vi "subAxisParamEx.vi"(1 "AxisId":i32=1, 2 "Index":i32=1) -> ()   [LabVIEW 2020]
panel:
  in  "SetOne":bool
  in  "PwmFreq":u16(ring) caption="Pwm frequency [Hz]" items=["20000", "80000"]
  in  "EncLines":i32=500 caption="Encoder lines" min=1 max=65535
  in  "MotorCommCounts":i32=1 caption="Encoder counts per commutating cycle" min=1 max=65535
  in  "PhaseInitAmp":i32 caption="Phase init. amplitude" min=0 max=100
  in  "MotorPoles":i32=1 caption="Motor poles" min=1 max=65535
  in  "MicrostepMode":i32=1 caption="Microstep mode" min=1 max=256
  in  "HoldCur":i32 caption="Hold current [%]" min=0 max=100
  in  "BrakeDecel":dbl caption="Brake deceleration" min=0.0 format="%.3f"
  in  "Vel":dbl format="%.3f"
  in  "RefDecel":dbl caption="Deceleration" min=0.0 format="%.3f"
  in  "SlowRefVel":dbl caption="Slow velocity [mm/s]" max=16777215.0 format="%.3f"
  in  "Jerk":i32 min=0
  in  "Decel":dbl caption="Deceleration" min=0.0 format="%.3f"
  in  "PhaseInitTime":i32=1 caption="Phase init. time" min=0
  in  "DriveCur":i32 caption="Drive current [%]" min=0 max=100
  in  "MaxPosErr":i32=10000 caption="Max. pos. error [Inc]" min=0
  in  "SampleTime":i32=256 caption="Sample time [µs]" min=204 max=19968
  in  "MaxOut":i32=99 caption="Maximum output [%]" min=0 max=99
  out "SetNr":u8
  in  "KD":i32=150
  in  "I-Limit":i32=100000
  in  "KI":i32=20
  in  "D-Time":i32 caption="Time"
  in  "KP":i32=30
  in  "Accel":dbl caption="Acceleration" format="%.3f"
  in  "FastRefVel":dbl caption="Fast velocity [mm/s]" max=16777215.0 format="%.3f"
  in  "FreeVel":dbl caption="Free velocity [mm/s]" min=0.0 max=16777215.0 format="%.3f"
  in  "PosVel":dbl caption="Velocity [mm/s]" max=16777215.0 format="%.3f"
  in  "SetAll":bool
  in  "End":bool
  # "Axis"
  # "Positioning"
  # "Reference run"
  # "Limit switches"
  # "Power amplifier"
  # "Velocity mode"
  # "[mm/s]"
  # "PID regulator"
  # "Step motor data"
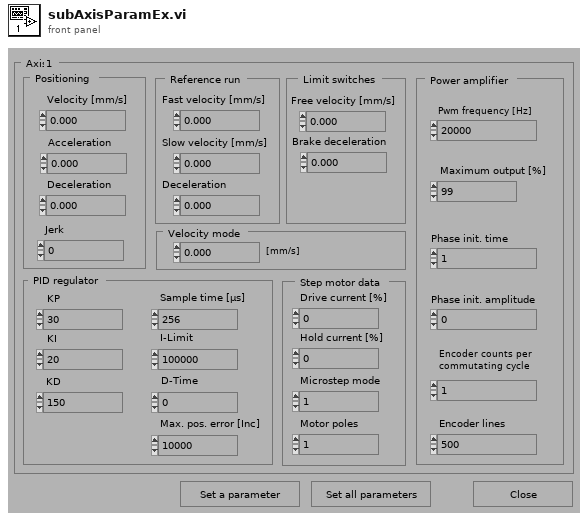
[diagram p1: front panel]
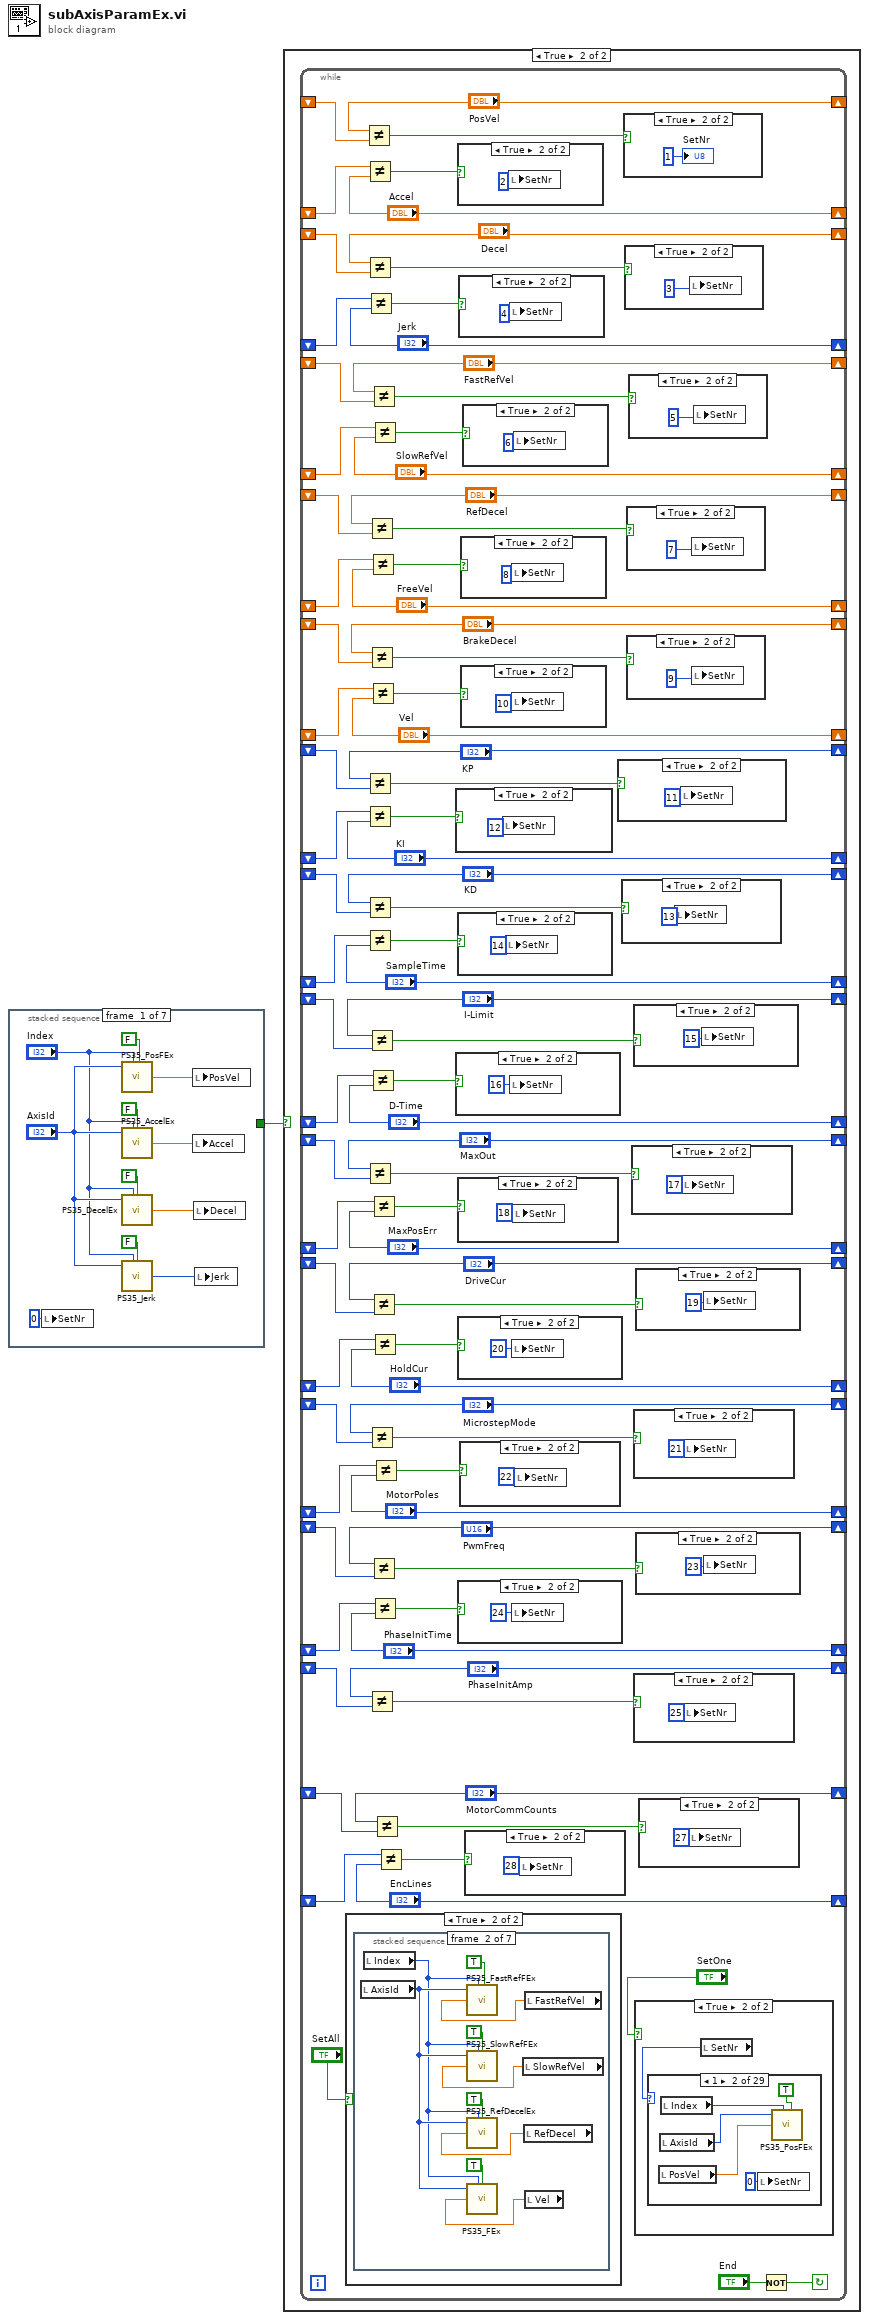
[diagram p0: block diagram]
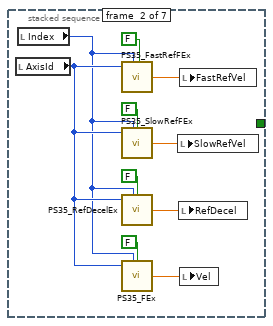
[diagram p2: hidden frame]
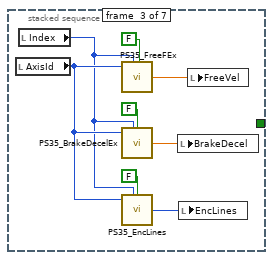
[diagram p3: hidden frame]
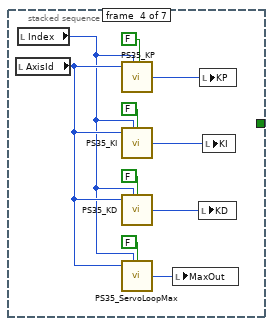
[diagram p4: hidden frame]
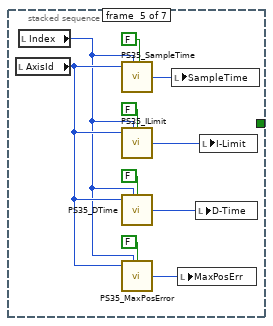
[diagram p5: hidden frame]
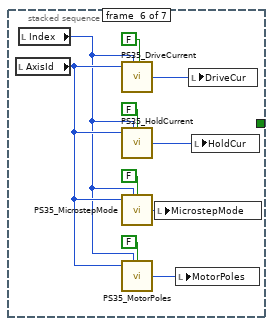
[diagram p6: hidden frame]
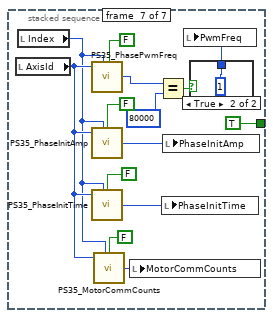
[diagram p7: hidden frame]
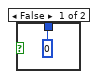
[diagram p8: hidden frame]
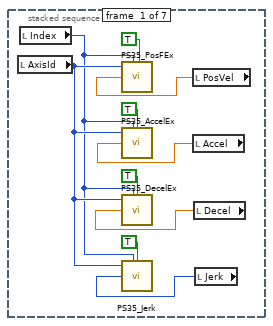
[diagram p11: hidden frame]
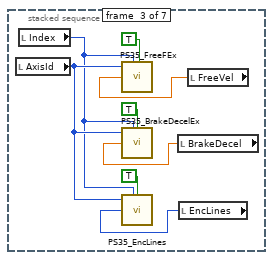
[diagram p12: hidden frame]
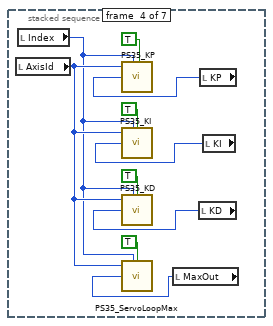
[diagram p13: hidden frame]
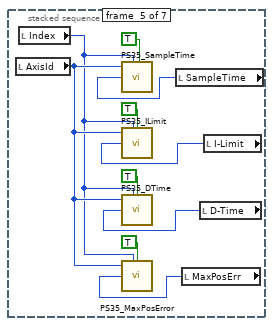
[diagram p14: hidden frame]
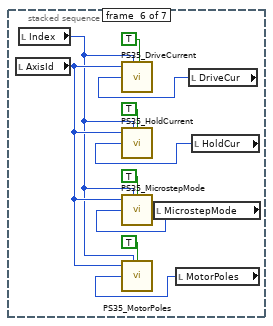
[diagram p15: hidden frame]
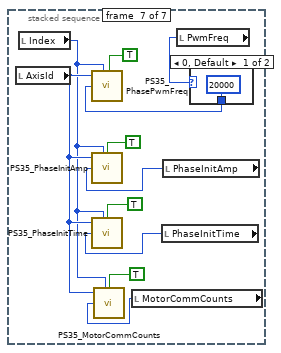
[diagram p16: hidden frame]
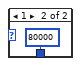
[diagram p17: hidden frame]
diagram:
  n1 = stacked-sequence {
    tunnel: [_ _ _ _ _ _ TRUE] -> w1
    frame #0 {
      n2 = local write "SetNr"(u8 0 ("SetNr")) -> ()
      n3 = call "PS35_PosFEx.vi"("Axis number"="AxisId", "Control unit ID"="Index", "function"=FALSE ("WriteRead")) -> ("dValue-Out"=w10:dbl)  [unwired: 5 in, 1 out]
      n4 = call "PS35_AccelEx.vi"("Axis number"="AxisId", "Control unit ID"="Index", "function"=FALSE ("WriteRead")) -> ("dValue-Out"=w9:dbl)  [unwired: 5 in, 1 out]
      n5 = call "PS35_DecelEx.vi"("Axis number"="AxisId", "Control unit ID"="Index", "function"=FALSE ("WriteRead")) -> ("dValue-Out"=w6:dbl)  [unwired: 5 in, 1 out]
      n6 = call "PS35_Jerk.vi"("Axis number"="AxisId", "Control unit ID"="Index", "function"=FALSE ("WriteRead")) -> ("Value-Out"=w5:i32)  [unwired: 5 in, 1 out]
      n7 = local write "PosVel"(w10) -> ()
      n8 = local write "Accel"(w9) -> ()
      n9 = local write "Decel"(w6) -> ()
      n10 = local write "Jerk"(w5) -> ()
    }
    frame #1 {
      n11 = local read "AxisId"() -> (w14:i32)
      n12 = local read "Index"() -> (w13:i32)
      n13 = call "PS35_FastRefFEx.vi"("Axis number"=w14, "Control unit ID"=w13, "function"=FALSE ("WriteRead")) -> ("dValue-Out"=w21:dbl)  [unwired: 5 in, 1 out]
      n14 = call "PS35_SlowRefFEx.vi"("Axis number"=w14, "Control unit ID"=w13, "function"=FALSE ("WriteRead")) -> ("dValue-Out"=w20:dbl)  [unwired: 5 in, 1 out]
      n15 = call "PS35_RefDecelEx.vi"("Axis number"=w14, "Control unit ID"=w13, "function"=FALSE ("WriteRead")) -> ("dValue-Out"=w17:dbl)  [unwired: 5 in, 1 out]
      n16 = call "PS35_FEx.vi"("Axis number"=w14, "Control unit ID"=w13, "function"=FALSE ("WriteRead")) -> ("dValue-Out"=w16:dbl)  [unwired: 5 in, 1 out]
      n17 = local write "SlowRefVel"(w20) -> ()
      n18 = local write "RefDecel"(w17) -> ()
      n19 = local write "FastRefVel"(w21) -> ()
      n20 = local write "Vel"(w16) -> ()
    }
    frame #2 {
      n21 = local read "AxisId"() -> (w24:i32)
      n22 = local read "Index"() -> (w23:i32)
      n23 = call "PS35_FreeFEx.vi"("Axis number"=w24, "Control unit ID"=w23, "function"=FALSE ("WriteRead")) -> ("dValue-Out"=w29:dbl)  [unwired: 5 in, 1 out]
      n24 = call "PS35_BrakeDecelEx.vi"("Axis number"=w24, "Control unit ID"=w23, "function"=FALSE ("WriteRead")) -> ("dValue-Out"=w28:dbl)  [unwired: 5 in, 1 out]
      n25 = call "PS35_EncLines.vi"("Axis number"=w24, "Control unit ID"=w23, "function"=FALSE ("WriteRead")) -> ("Value-Out"=w25:i32)  [unwired: 5 in, 1 out]
      n26 = local write "BrakeDecel"(w28) -> ()
      n27 = local write "EncLines"(w25) -> ()
      n28 = local write "FreeVel"(w29) -> ()
    }
    frame #3 {
      n29 = local read "AxisId"() -> (w32:i32)
      n30 = local read "Index"() -> (w31:i32)
      n31 = call "PS35_KP.vi"("Axis number"=w32, "Control unit ID"=w31, "function"=FALSE ("WriteRead")) -> ("Value-Out"=w39:i32)  [unwired: 5 in, 1 out]
      n32 = call "PS35_KI.vi"("Axis number"=w32, "Control unit ID"=w31, "function"=FALSE ("WriteRead")) -> ("Value-Out"=w38:i32)  [unwired: 5 in, 1 out]
      n33 = call "PS35_KD.vi"("Axis number"=w32, "Control unit ID"=w31, "function"=FALSE ("WriteRead")) -> ("Value-Out"=w35:i32)  [unwired: 5 in, 1 out]
      n34 = call "PS35_ServoLoopMax.vi"("Axis number"=w32, "Control unit ID"=w31, "function"=FALSE ("WriteRead")) -> ("Value-Out"=w34:i32)  [unwired: 5 in, 1 out]
      n35 = local write "MaxOut"(w34) -> ()
      n36 = local write "KD"(w35) -> ()
      n37 = local write "KP"(w39) -> ()
      n38 = local write "KI"(w38) -> ()
    }
    frame #4 {
      n39 = local read "AxisId"() -> (w42:i32)
      n40 = local read "Index"() -> (w41:i32)
      n41 = call "PS35_SampleTime.vi"("Axis number"=w42, "Control unit ID"=w41, "function"=FALSE ("WriteRead")) -> ("Value-Out"=w49:i32)  [unwired: 5 in, 1 out]
      n42 = call "PS35_ILimit.vi"("Axis number"=w42, "Control unit ID"=w41, "function"=FALSE ("WriteRead")) -> ("Value-Out"=w48:i32)  [unwired: 5 in, 1 out]
      n43 = call "PS35_DTime.vi"("Axis number"=w42, "Control unit ID"=w41, "function"=FALSE ("WriteRead")) -> ("Value-Out"=w45:i32)  [unwired: 5 in, 1 out]
      n44 = call "PS35_MaxPosError.vi"("Axis number"=w42, "Control unit ID"=w41, "function"=FALSE ("WriteRead")) -> ("Value-Out"=w44:i32)  [unwired: 5 in, 1 out]
      n45 = local write "SampleTime"(w49) -> ()
      n46 = local write "MaxPosErr"(w44) -> ()
      n47 = local write "D-Time"(w45) -> ()
      n48 = local write "I-Limit"(w48) -> ()
    }
    frame #5 {
      n49 = local read "AxisId"() -> (w52:i32)
      n50 = local read "Index"() -> (w51:i32)
      n51 = call "PS35_DriveCurrent.vi"("Axis number"=w52, "Control unit ID"=w51, "function"=FALSE ("WriteRead")) -> ("Value-Out"=w59:i32)  [unwired: 5 in, 1 out]
      n52 = call "PS35_HoldCurrent.vi"("Axis number"=w52, "Control unit ID"=w51, "function"=FALSE ("WriteRead")) -> ("Value-Out"=w58:i32)  [unwired: 5 in, 1 out]
      n53 = call "PS35_MicrostepMode.vi"("Axis number"=w52, "Control unit ID"=w51, "function"=FALSE ("WriteRead")) -> ("Value-Out"=w55:i32)  [unwired: 5 in, 1 out]
      n54 = call "PS35_MotorPoles.vi"("Axis number"=w52, "Control unit ID"=w51, "function"=FALSE ("WriteRead")) -> ("Value-Out"=w54:i32)  [unwired: 5 in, 1 out]
      n55 = local write "MicrostepMode"(w55) -> ()
      n56 = local write "MotorPoles"(w54) -> ()
      n57 = local write "DriveCur"(w59) -> ()
      n58 = local write "HoldCur"(w58) -> ()
    }
    frame #6 {
      n59 = local read "AxisId"() -> (w62:i32)
      n60 = local read "Index"() -> (w61:i32)
      n61 = call "PS35_PhasePwmFreq.vi"("Axis number"=w62, "Control unit ID"=w61, "function"=FALSE ("WriteRead")) -> ("Value-Out"=w66:i32)  [unwired: 5 in, 1 out]
      n62 = call "PS35_PhaseInitAmp.vi"("Axis number"=w62, "Control unit ID"=w61, "function"=FALSE ("WriteRead")) -> ("Value-Out"=w73:i32)  [unwired: 5 in, 1 out]
      n63 = call "PS35_PhaseInitTime.vi"("Axis number"=w62, "Control unit ID"=w61, "function"=FALSE ("WriteRead")) -> ("Value-Out"=w70:i32)  [unwired: 5 in, 1 out]
      n64 = call "PS35_MotorCommCounts.vi"("Axis number"=w62, "Control unit ID"=w61, "function"=FALSE ("WriteRead")) -> ("Value-Out"=w67:i32)  [unwired: 5 in, 1 out]
      n65 = local write "MotorCommCounts"(w67) -> ()
      n66 = Equal?(x=w66, y=80000) -> (x = y?=w64:bool)
      n67 = local write "PhaseInitTime"(w70) -> ()
      n68 = local write "PhaseInitAmp"(w73) -> ()
      n69 = case shown="True" w64 {
        tunnel: [0 1] -> w63
        frame False {
        }
        frame True {
        }
      }
      n70 = local write "PwmFreq"(w63) -> ()
    }
  }
  n71 = case shown="True" w1 {
    frame False {
    }
    frame True {
      n72 = while {
        shift-left: _ -> [w81]
        shift-right: ["EncLines"] -> _
        shift-left: _ -> [w83]
        shift-right: ["MotorCommCounts"] -> _
        shift-left: _ -> [w88]
        shift-right: ["PhaseInitTime"] -> _
        shift-left: _ -> [w90]
        shift-right: ["PwmFreq"] -> _
        shift-left: _ -> [w91]
        shift-right: ["PhaseInitAmp"] -> _
        shift-left: _ -> [w103]
        shift-right: ["HoldCur"] -> _
        shift-left: _ -> [w101]
        shift-right: ["DriveCur"] -> _
        shift-left: _ -> [w98]
        shift-right: ["MotorPoles"] -> _
        shift-left: _ -> [w100]
        shift-right: ["MicrostepMode"] -> _
        shift-left: _ -> [w114]
        shift-right: ["BrakeDecel"] -> _
        shift-left: _ -> [w116]
        shift-right: ["Vel"] -> _
        shift-left: _ -> [w123]
        shift-right: ["RefDecel"] -> _
        shift-left: _ -> [w121]
        shift-right: ["FreeVel"] -> _
        shift-left: _ -> [w126]
        shift-right: ["FastRefVel"] -> _
        shift-left: _ -> [w128]
        shift-right: ["SlowRefVel"] -> _
        shift-left: _ -> [w133]
        shift-right: ["Decel"] -> _
        shift-left: _ -> [w131]
        shift-right: ["Jerk"] -> _
        shift-left: _ -> [w138]
        shift-right: ["PosVel"] -> _
        shift-left: _ -> [w142]
        shift-right: ["D-Time"] -> _
        shift-left: _ -> [w144]
        shift-right: ["I-Limit"] -> _
        shift-left: _ -> [w148]
        shift-right: ["MaxPosErr"] -> _
        shift-left: _ -> [w146]
        shift-right: ["MaxOut"] -> _
        shift-left: _ -> [w151]
        shift-right: ["SampleTime"] -> _
        shift-left: _ -> [w153]
        shift-right: ["KD"] -> _
        shift-left: _ -> [w156]
        shift-right: ["KI"] -> _
        shift-left: _ -> [w154]
        shift-right: ["KP"] -> _
        shift-left: _ -> [w159]
        shift-right: ["Accel"] -> _
        stop <- w161 continue-if-true
        n73 = case shown="True" "SetAll" {
          frame False {
          }
          frame True {
            n74 = stacked-sequence {
              frame #0 {
                n75 = local read "AxisId"() -> (w164:i32)
                n76 = local read "Index"() -> (w162:i32)
                n77 = local read "PosVel"() -> (w167:dbl)
                n78 = call "PS35_PosFEx.vi"("Axis number"=w164, "Control unit ID"=w162, "dValue-In"=w167, "function"=TRUE ("WriteRead")) -> ()  [unwired: 4 in, 2 out]
                n79 = local read "Accel"() -> (w166:dbl)
                n80 = call "PS35_AccelEx.vi"("Axis number"=w164, "Control unit ID"=w162, "dValue-In"=w166, "function"=TRUE ("WriteRead")) -> ()  [unwired: 4 in, 2 out]
                n81 = local read "Decel"() -> (w165:dbl)
                n82 = call "PS35_DecelEx.vi"("Axis number"=w164, "Control unit ID"=w162, "dValue-In"=w165, "function"=TRUE ("WriteRead")) -> ()  [unwired: 4 in, 2 out]
                n83 = local read "Jerk"() -> (w163:i32)
                n84 = call "PS35_Jerk.vi"("Axis number"=w164, "Control unit ID"=w162, "Value-In"=w163, "function"=TRUE ("WriteRead")) -> ()  [unwired: 4 in, 2 out]
              }
              frame #1 {
                n85 = local read "AxisId"() -> (w177:i32)
                n86 = local read "Index"() -> (w172:i32)
                n87 = local read "SlowRefVel"() -> (w175:dbl)
                n88 = call "PS35_SlowRefFEx.vi"("Axis number"=w177, "Control unit ID"=w172, "dValue-In"=w175, "function"=TRUE ("WriteRead")) -> ()  [unwired: 4 in, 2 out]
                n89 = local read "RefDecel"() -> (w174:dbl)
                n90 = call "PS35_RefDecelEx.vi"("Axis number"=w177, "Control unit ID"=w172, "dValue-In"=w174, "function"=TRUE ("WriteRead")) -> ()  [unwired: 4 in, 2 out]
                n91 = local read "FastRefVel"() -> (w176:dbl)
                n92 = call "PS35_FastRefFEx.vi"("Axis number"=w177, "Control unit ID"=w172, "dValue-In"=w176, "function"=TRUE ("WriteRead")) -> ()  [unwired: 4 in, 2 out]
                n93 = local read "Vel"() -> (w173:dbl)
                n94 = call "PS35_FEx.vi"("Axis number"=w177, "Control unit ID"=w172, "dValue-In"=w173, "function"=TRUE ("WriteRead")) -> ()  [unwired: 4 in, 2 out]
              }
              frame #2 {
                n95 = local read "AxisId"() -> (w186:i32)
                n96 = local read "Index"() -> (w182:i32)
                n97 = local read "BrakeDecel"() -> (w184:dbl)
                n98 = call "PS35_BrakeDecelEx.vi"("Axis number"=w186, "Control unit ID"=w182, "dValue-In"=w184, "function"=TRUE ("WriteRead")) -> ()  [unwired: 4 in, 2 out]
                n99 = local read "EncLines"() -> (w183:i32)
                n100 = call "PS35_EncLines.vi"("Axis number"=w186, "Control unit ID"=w182, "Value-In"=w183, "function"=TRUE ("WriteRead")) -> ()  [unwired: 4 in, 2 out]
                n101 = local read "FreeVel"() -> (w185:dbl)
                n102 = call "PS35_FreeFEx.vi"("Axis number"=w186, "Control unit ID"=w182, "dValue-In"=w185, "function"=TRUE ("WriteRead")) -> ()  [unwired: 4 in, 2 out]
              }
              frame #3 {
                n103 = local read "AxisId"() -> (w195:i32)
                n104 = local read "Index"() -> (w190:i32)
                n105 = local read "MaxOut"() -> (w191:i32)
                n106 = call "PS35_ServoLoopMax.vi"("Axis number"=w195, "Control unit ID"=w190, "Value-In"=w191, "function"=TRUE ("WriteRead")) -> ()  [unwired: 4 in, 2 out]
                n107 = local read "KD"() -> (w192:i32)
                n108 = call "PS35_KD.vi"("Axis number"=w195, "Control unit ID"=w190, "Value-In"=w192, "function"=TRUE ("WriteRead")) -> ()  [unwired: 4 in, 2 out]
                n109 = local read "KP"() -> (w194:i32)
                n110 = call "PS35_KP.vi"("Axis number"=w195, "Control unit ID"=w190, "Value-In"=w194, "function"=TRUE ("WriteRead")) -> ()  [unwired: 4 in, 2 out]
                n111 = local read "KI"() -> (w193:i32)
                n112 = call "PS35_KI.vi"("Axis number"=w195, "Control unit ID"=w190, "Value-In"=w193, "function"=TRUE ("WriteRead")) -> ()  [unwired: 4 in, 2 out]
              }
              frame #4 {
                n113 = local read "AxisId"() -> (w205:i32)
                n114 = local read "Index"() -> (w200:i32)
                n115 = local read "SampleTime"() -> (w204:i32)
                n116 = call "PS35_SampleTime.vi"("Axis number"=w205, "Control unit ID"=w200, "Value-In"=w204, "function"=TRUE ("WriteRead")) -> ()  [unwired: 4 in, 2 out]
                n117 = local read "MaxPosErr"() -> (w201:i32)
                n118 = call "PS35_MaxPosError.vi"("Axis number"=w205, "Control unit ID"=w200, "Value-In"=w201, "function"=TRUE ("WriteRead")) -> ()  [unwired: 4 in, 2 out]
                n119 = local read "D-Time"() -> (w202:i32)
                n120 = call "PS35_DTime.vi"("Axis number"=w205, "Control unit ID"=w200, "Value-In"=w202, "function"=TRUE ("WriteRead")) -> ()  [unwired: 4 in, 2 out]
                n121 = local read "I-Limit"() -> (w203:i32)
                n122 = call "PS35_ILimit.vi"("Axis number"=w205, "Control unit ID"=w200, "Value-In"=w203, "function"=TRUE ("WriteRead")) -> ()  [unwired: 4 in, 2 out]
              }
              frame #5 {
                n123 = local read "AxisId"() -> (w215:i32)
                n124 = local read "Index"() -> (w210:i32)
                n125 = local read "MicrostepMode"() -> (w212:i32)
                n126 = call "PS35_MicrostepMode.vi"("Axis number"=w215, "Control unit ID"=w210, "Value-In"=w212, "function"=TRUE ("WriteRead")) -> ()  [unwired: 4 in, 2 out]
                n127 = local read "MotorPoles"() -> (w211:i32)
                n128 = call "PS35_MotorPoles.vi"("Axis number"=w215, "Control unit ID"=w210, "Value-In"=w211, "function"=TRUE ("WriteRead")) -> ()  [unwired: 4 in, 2 out]
                n129 = local read "DriveCur"() -> (w214:i32)
                n130 = call "PS35_DriveCurrent.vi"("Axis number"=w215, "Control unit ID"=w210, "Value-In"=w214, "function"=TRUE ("WriteRead")) -> ()  [unwired: 4 in, 2 out]
                n131 = local read "HoldCur"() -> (w213:i32)
                n132 = call "PS35_HoldCurrent.vi"("Axis number"=w215, "Control unit ID"=w210, "Value-In"=w213, "function"=TRUE ("WriteRead")) -> ()  [unwired: 4 in, 2 out]
              }
              frame #6 {
                n133 = local read "AxisId"() -> (w222:i32)
                n134 = local read "Index"() -> (w220:i32)
                n135 = local read "MotorCommCounts"() -> (w221:i32)
                n136 = call "PS35_MotorCommCounts.vi"("Axis number"=w222, "Control unit ID"=w220, "Value-In"=w221, "function"=TRUE ("WriteRead")) -> ()  [unwired: 4 in, 2 out]
                n137 = local read "PhaseInitTime"() -> (w223:i32)
                n138 = call "PS35_PhaseInitTime.vi"("Axis number"=w222, "Control unit ID"=w220, "Value-In"=w223, "function"=TRUE ("WriteRead")) -> ()  [unwired: 4 in, 2 out]
                n139 = local read "PhaseInitAmp"() -> (w224:i32)
                n140 = call "PS35_PhaseInitAmp.vi"("Axis number"=w222, "Control unit ID"=w220, "Value-In"=w224, "function"=TRUE ("WriteRead")) -> ()  [unwired: 4 in, 2 out]
                n141 = local read "PwmFreq"() -> (w226:u16)
                n142 = case shown="0, Default" w226 {
                  tunnel: [20000 80000] -> w225
                  frame 0, Default {
                  }
                  frame 1 {
                  }
                }
                n143 = call "PS35_PhasePwmFreq.vi"("Axis number"=w222, "Control unit ID"=w220, "Value-In"=w225, "function"=TRUE ("WriteRead")) -> ()  [unwired: 4 in, 2 out]
              }
            }
          }
        }
        n144 = Not Equal?(x="PosVel", y=w138) -> (x != y?=w137:bool)
        n145 = Not Equal?(x=w159, y="Accel") -> (x != y?=w158:bool)
        n146 = Not Equal?(x="Decel", y=w133) -> (x != y?=w134:bool)
        n147 = Not Equal?(x="KP", y=w154) -> (x != y?=w155:bool)
        n148 = Not Equal?(x=w156, y="KI") -> (x != y?=w157:bool)
        n149 = Not Equal?(x="KD", y=w153) -> (x != y?=w152:bool)
        n150 = Not Equal?(x=w151, y="SampleTime") -> (x != y?=w150:bool)
        n151 = Not Equal?(x="MaxOut", y=w146) -> (x != y?=w147:bool)
        n152 = Not Equal?(x=w131, y="Jerk") -> (x != y?=w132:bool)
        n153 = Not Equal?(x="RefDecel", y=w123) -> (x != y?=w124:bool)
        n154 = Not Equal?(x="BrakeDecel", y=w114) -> (x != y?=w113:bool)
        n155 = Not Equal?(x="I-Limit", y=w144) -> (x != y?=w143:bool)
        n156 = Not Equal?(x="MicrostepMode", y=w100) -> (x != y?=w99:bool)
        n157 = Not Equal?(x="PhaseInitAmp", y=w91) -> (x != y?=w92:bool)
        n158 = Not Equal?(x=w121, y="FreeVel") -> (x != y?=w122:bool)
        n159 = Not Equal?(x=w116, y="Vel") -> (x != y?=w115:bool)
        n160 = Not Equal?(x=w142, y="D-Time") -> (x != y?=w141:bool)
        n161 = Not Equal?(x="FastRefVel", y=w126) -> (x != y?=w125:bool)
        n162 = Not Equal?(x=w148, y="MaxPosErr") -> (x != y?=w149:bool)
        n163 = Not Equal?(x="DriveCur", y=w101) -> (x != y?=w102:bool)
        n164 = Not Equal?(x="PwmFreq", y=w90) -> (x != y?=w89:bool)
        n165 = Not Equal?(x=w128, y="SlowRefVel") -> (x != y?=w127:bool)
        n166 = Not Equal?(x=w103, y="HoldCur") -> (x != y?=w104:bool)
        n167 = Not Equal?(x=w88, y="PhaseInitTime") -> (x != y?=w87:bool)
        n168 = Not Equal?(x=w98, y="MotorPoles") -> (x != y?=w97:bool)
        n169 = Not Equal?(x="MotorCommCounts", y=w83) -> (x != y?=w82:bool)
        n170 = Not Equal?(x=w81, y="EncLines") -> (x != y?=w80:bool)
        n171 = case shown="True" w157 {
          frame False {
          }
          frame True {
            n172 = local write "SetNr"(u8 12 ("SetNr")) -> ()
          }
        }
        n173 = case shown="True" w141 {
          frame False {
          }
          frame True {
            n174 = local write "SetNr"(u8 16 ("SetNr")) -> ()
          }
        }
        n175 = case shown="True" w158 {
          frame False {
          }
          frame True {
            n176 = local write "SetNr"(u8 2 ("SetNr")) -> ()
          }
        }
        n177 = case shown="True" w150 {
          frame False {
          }
          frame True {
            n178 = local write "SetNr"(u8 14 ("SetNr")) -> ()
          }
        }
        n179 = case shown="True" w149 {
          frame False {
          }
          frame True {
            n180 = local write "SetNr"(u8 18 ("SetNr")) -> ()
          }
        }
        n181 = case shown="True" w104 {
          frame False {
          }
          frame True {
            n182 = local write "SetNr"(u8 20 ("SetNr")) -> ()
          }
        }
        n183 = case shown="True" w87 {
          frame False {
          }
          frame True {
            n184 = local write "SetNr"(u8 24 ("SetNr")) -> ()
          }
        }
        n185 = case shown="True" w132 {
          frame False {
          }
          frame True {
            n186 = local write "SetNr"(u8 4 ("SetNr")) -> ()
          }
        }
        n187 = case shown="True" w97 {
          frame False {
          }
          frame True {
            n188 = local write "SetNr"(u8 22 ("SetNr")) -> ()
          }
        }
        n189 = case shown="True" w122 {
          frame False {
          }
          frame True {
            n190 = local write "SetNr"(u8 8 ("SetNr")) -> ()
          }
        }
        n191 = case shown="True" w115 {
          frame False {
          }
          frame True {
            n192 = local write "SetNr"(u8 10 ("SetNr")) -> ()
          }
        }
        n193 = case shown="True" w127 {
          frame False {
          }
          frame True {
            n194 = local write "SetNr"(u8 6 ("SetNr")) -> ()
          }
        }
        n195 = case shown="True" w80 {
          frame False {
          }
          frame True {
            n196 = local write "SetNr"(u8 28 ("SetNr")) -> ()
          }
        }
        n197 = case shown="True" w155 {
          frame False {
          }
          frame True {
            n198 = local write "SetNr"(u8 11 ("SetNr")) -> ()
          }
        }
        n199 = case shown="True" w152 {
          frame False {
          }
          frame True {
            n200 = local write "SetNr"(u8 13 ("SetNr")) -> ()
          }
        }
        n201 = case shown="True" w137 {
          frame False {
          }
          frame True {
            "SetNr" <- u8 1 ("SetNr")
          }
        }
        n202 = case shown="True" w134 {
          frame False {
          }
          frame True {
            n203 = local write "SetNr"(u8 3 ("SetNr")) -> ()
          }
        }
        n204 = case shown="True" w124 {
          frame False {
          }
          frame True {
            n205 = local write "SetNr"(u8 7 ("SetNr")) -> ()
          }
        }
        n206 = case shown="True" w113 {
          frame False {
          }
          frame True {
            n207 = local write "SetNr"(u8 9 ("SetNr")) -> ()
          }
        }
        n208 = case shown="True" w125 {
          frame False {
          }
          frame True {
            n209 = local write "SetNr"(u8 5 ("SetNr")) -> ()
          }
        }
        n210 = case shown="True" w147 {
          frame False {
          }
          frame True {
            n211 = local write "SetNr"(u8 17 ("SetNr")) -> ()
          }
        }
        n212 = case shown="True" w143 {
          frame False {
          }
          frame True {
            n213 = local write "SetNr"(u8 15 ("SetNr")) -> ()
          }
        }
        n214 = case shown="True" w99 {
          frame False {
          }
          frame True {
            n215 = local write "SetNr"(u8 21 ("SetNr")) -> ()
          }
        }
        n216 = case shown="True" w92 {
          frame False {
          }
          frame True {
            n217 = local write "SetNr"(u8 25 ("SetNr")) -> ()
          }
        }
        n218 = case shown="True" "SetOne" {
          frame False {
          }
          frame True {
            n219 = local read "SetNr"() -> (w260:u8)
            n220 = case shown="1" w260 {
              frame 0, Default {
              }
              frame 1 {
                n221 = local read "PosVel"() -> (w262:dbl)
                n222 = local read "AxisId"() -> (w263:i32)
                n223 = local read "Index"() -> (w261:i32)
                n224 = local write "SetNr"(u8 0 ("SetNr")) -> ()
                n225 = call "PS35_PosFEx.vi"("Axis number"=w263, "Control unit ID"=w261, "dValue-In"=w262, "function"=TRUE ("WriteRead")) -> ()  [unwired: 4 in, 2 out]
              }
              frame 2 {
                n226 = local read "AxisId"() -> (w268:i32)
                n227 = local read "Index"() -> (w266:i32)
                n228 = local read "Accel"() -> (w267:dbl)
                n229 = local write "SetNr"(u8 0 ("SetNr")) -> ()
                n230 = call "PS35_AccelEx.vi"("Axis number"=w268, "Control unit ID"=w266, "dValue-In"=w267, "function"=TRUE ("WriteRead")) -> ()  [unwired: 4 in, 2 out]
              }
              frame 3 {
                n231 = local read "AxisId"() -> (w273:i32)
                n232 = local read "Decel"() -> (w272:dbl)
                n233 = local read "Index"() -> (w271:i32)
                n234 = local write "SetNr"(u8 0 ("SetNr")) -> ()
                n235 = call "PS35_DecelEx.vi"("Axis number"=w273, "Control unit ID"=w271, "dValue-In"=w272, "function"=TRUE ("WriteRead")) -> ()  [unwired: 4 in, 2 out]
              }
              frame 4 {
                n236 = local read "AxisId"() -> (w278:i32)
                n237 = local read "Index"() -> (w276:i32)
                n238 = local read "Jerk"() -> (w277:i32)
                n239 = local write "SetNr"(u8 0 ("SetNr")) -> ()
                n240 = call "PS35_Jerk.vi"("Axis number"=w278, "Control unit ID"=w276, "Value-In"=w277, "function"=TRUE ("WriteRead")) -> ()  [unwired: 4 in, 2 out]
              }
              frame 5 {
                n241 = local read "AxisId"() -> (w283:i32)
                n242 = local read "FastRefVel"() -> (w282:dbl)
                n243 = local read "Index"() -> (w281:i32)
                n244 = local write "SetNr"(u8 0 ("SetNr")) -> ()
                n245 = call "PS35_FastRefFEx.vi"("Axis number"=w283, "Control unit ID"=w281, "dValue-In"=w282, "function"=TRUE ("WriteRead")) -> ()  [unwired: 4 in, 2 out]
              }
              frame 6 {
                n246 = local read "SlowRefVel"() -> (w287:dbl)
                n247 = local read "AxisId"() -> (w288:i32)
                n248 = local read "Index"() -> (w286:i32)
                n249 = local write "SetNr"(u8 0 ("SetNr")) -> ()
                n250 = call "PS35_SlowRefFEx.vi"("Axis number"=w288, "Control unit ID"=w286, "dValue-In"=w287, "function"=TRUE ("WriteRead")) -> ()  [unwired: 4 in, 2 out]
              }
              frame 7 {
                n251 = local read "AxisId"() -> (w293:i32)
                n252 = local read "RefDecel"() -> (w292:dbl)
                n253 = local read "Index"() -> (w291:i32)
                n254 = local write "SetNr"(u8 0 ("SetNr")) -> ()
                n255 = call "PS35_RefDecelEx.vi"("Axis number"=w293, "Control unit ID"=w291, "dValue-In"=w292, "function"=TRUE ("WriteRead")) -> ()  [unwired: 4 in, 2 out]
              }
              frame 8 {
                n256 = local read "AxisId"() -> (w298:i32)
                n257 = local read "Index"() -> (w296:i32)
                n258 = local read "FreeVel"() -> (w297:dbl)
                n259 = local write "SetNr"(u8 0 ("SetNr")) -> ()
                n260 = call "PS35_FreeFEx.vi"("Axis number"=w298, "Control unit ID"=w296, "dValue-In"=w297, "function"=TRUE ("WriteRead")) -> ()  [unwired: 4 in, 2 out]
              }
              frame 9 {
                n261 = local read "BrakeDecel"() -> (w302:dbl)
                n262 = local read "AxisId"() -> (w303:i32)
                n263 = local read "Index"() -> (w301:i32)
                n264 = local write "SetNr"(u8 0 ("SetNr")) -> ()
                n265 = call "PS35_BrakeDecelEx.vi"("Axis number"=w303, "Control unit ID"=w301, "dValue-In"=w302, "function"=TRUE ("WriteRead")) -> ()  [unwired: 4 in, 2 out]
              }
              frame 10 {
                n266 = local read "AxisId"() -> (w308:i32)
                n267 = local read "Index"() -> (w306:i32)
                n268 = local read "Vel"() -> (w307:dbl)
                n269 = local write "SetNr"(u8 0 ("SetNr")) -> ()
                n270 = call "PS35_FEx.vi"("Axis number"=w308, "Control unit ID"=w306, "dValue-In"=w307, "function"=TRUE ("WriteRead")) -> ()  [unwired: 4 in, 2 out]
              }
              frame 11 {
                n271 = local read "AxisId"() -> (w313:i32)
                n272 = local read "Index"() -> (w311:i32)
                n273 = local read "KP"() -> (w312:i32)
                n274 = local write "SetNr"(u8 0 ("SetNr")) -> ()
                n275 = call "PS35_KP.vi"("Axis number"=w313, "Control unit ID"=w311, "Value-In"=w312, "function"=TRUE ("WriteRead")) -> ()  [unwired: 4 in, 2 out]
              }
              frame 12 {
                n276 = local read "AxisId"() -> (w318:i32)
                n277 = local read "Index"() -> (w316:i32)
                n278 = local read "KI"() -> (w317:i32)
                n279 = local write "SetNr"(u8 0 ("SetNr")) -> ()
                n280 = call "PS35_KI.vi"("Axis number"=w318, "Control unit ID"=w316, "Value-In"=w317, "function"=TRUE ("WriteRead")) -> ()  [unwired: 4 in, 2 out]
              }
              frame 13 {
                n281 = local read "AxisId"() -> (w323:i32)
                n282 = local read "Index"() -> (w321:i32)
                n283 = local read "KD"() -> (w322:i32)
                n284 = local write "SetNr"(u8 0 ("SetNr")) -> ()
                n285 = call "PS35_KD.vi"("Axis number"=w323, "Control unit ID"=w321, "Value-In"=w322, "function"=TRUE ("WriteRead")) -> ()  [unwired: 4 in, 2 out]
              }
              frame 14 {
                n286 = local read "SampleTime"() -> (w327:i32)
                n287 = local read "AxisId"() -> (w328:i32)
                n288 = local read "Index"() -> (w326:i32)
                n289 = local write "SetNr"(u8 0 ("SetNr")) -> ()
                n290 = call "PS35_SampleTime.vi"("Axis number"=w328, "Control unit ID"=w326, "Value-In"=w327, "function"=TRUE ("WriteRead")) -> ()  [unwired: 4 in, 2 out]
              }
              frame 15 {
                n291 = local read "I-Limit"() -> (w332:i32)
                n292 = local read "Index"() -> (w331:i32)
                n293 = local read "AxisId"() -> (w333:i32)
                n294 = local write "SetNr"(u8 0 ("SetNr")) -> ()
                n295 = call "PS35_ILimit.vi"("Axis number"=w333, "Control unit ID"=w331, "Value-In"=w332, "function"=TRUE ("WriteRead")) -> ()  [unwired: 4 in, 2 out]
              }
              frame 16 {
                n296 = local read "D-Time"() -> (w337:i32)
                n297 = local read "AxisId"() -> (w338:i32)
                n298 = local read "Index"() -> (w336:i32)
                n299 = local write "SetNr"(u8 0 ("SetNr")) -> ()
                n300 = call "PS35_DTime.vi"("Axis number"=w338, "Control unit ID"=w336, "Value-In"=w337, "function"=TRUE ("WriteRead")) -> ()  [unwired: 4 in, 2 out]
              }
              frame 17 {
                n301 = local read "MaxOut"() -> (w342:i32)
                n302 = local read "AxisId"() -> (w343:i32)
                n303 = local read "Index"() -> (w341:i32)
                n304 = local write "SetNr"(u8 0 ("SetNr")) -> ()
                n305 = call "PS35_ServoLoopMax.vi"("Axis number"=w343, "Control unit ID"=w341, "Value-In"=w342, "function"=TRUE ("WriteRead")) -> ()  [unwired: 4 in, 2 out]
              }
              frame 18 {
                n306 = local read "MaxPosErr"() -> (w347:i32)
                n307 = local read "AxisId"() -> (w348:i32)
                n308 = local read "Index"() -> (w346:i32)
                n309 = local write "SetNr"(u8 0 ("SetNr")) -> ()
                n310 = call "PS35_MaxPosError.vi"("Axis number"=w348, "Control unit ID"=w346, "Value-In"=w347, "function"=TRUE ("WriteRead")) -> ()  [unwired: 4 in, 2 out]
              }
              frame 19 {
                n311 = local read "AxisId"() -> (w353:i32)
                n312 = local read "DriveCur"() -> (w352:i32)
                n313 = local read "Index"() -> (w351:i32)
                n314 = local write "SetNr"(u8 0 ("SetNr")) -> ()
                n315 = call "PS35_DriveCurrent.vi"("Axis number"=w353, "Control unit ID"=w351, "Value-In"=w352, "function"=TRUE ("WriteRead")) -> ()  [unwired: 4 in, 2 out]
              }
              frame 20 {
                n316 = local read "HoldCur"() -> (w357:i32)
                n317 = local read "AxisId"() -> (w358:i32)
                n318 = local read "Index"() -> (w356:i32)
                n319 = local write "SetNr"(u8 0 ("SetNr")) -> ()
                n320 = call "PS35_HoldCurrent.vi"("Axis number"=w358, "Control unit ID"=w356, "Value-In"=w357, "function"=TRUE ("WriteRead")) -> ()  [unwired: 4 in, 2 out]
              }
              frame 21 {
                n321 = local read "MicrostepMode"() -> (w362:i32)
                n322 = local read "AxisId"() -> (w363:i32)
                n323 = local read "Index"() -> (w361:i32)
                n324 = local write "SetNr"(u8 0 ("SetNr")) -> ()
                n325 = call "PS35_MicrostepMode.vi"("Axis number"=w363, "Control unit ID"=w361, "Value-In"=w362, "function"=TRUE ("WriteRead")) -> ()  [unwired: 4 in, 2 out]
              }
              frame 22 {
                n326 = local read "MotorPoles"() -> (w367:i32)
                n327 = local read "AxisId"() -> (w368:i32)
                n328 = local read "Index"() -> (w366:i32)
                n329 = local write "SetNr"(u8 0 ("SetNr")) -> ()
                n330 = call "PS35_MotorPoles.vi"("Axis number"=w368, "Control unit ID"=w366, "Value-In"=w367, "function"=TRUE ("WriteRead")) -> ()  [unwired: 4 in, 2 out]
              }
              frame 23 {
                n331 = local read "AxisId"() -> (w374:i32)
                n332 = local read "PwmFreq"() -> (w373:u16)
                n333 = case shown="0, Default" w373 {
                  tunnel: [u32 20000 ("SetNr") u32 80000 ("SetNr")] -> w372
                  frame 0, Default {
                  }
                  frame 1 {
                  }
                }
                n334 = local read "Index"() -> (w371:i32)
                n335 = local write "SetNr"(u8 0 ("SetNr")) -> ()
                n336 = call "PS35_PhasePwmFreq.vi"("Axis number"=w374, "Control unit ID"=w371, "Value-In"=w372, "function"=TRUE ("WriteRead")) -> ()  [unwired: 4 in, 2 out]
              }
              frame 24 {
                n337 = local read "PhaseInitTime"() -> (w380:i32)
                n338 = local read "AxisId"() -> (w381:i32)
                n339 = local read "Index"() -> (w379:i32)
                n340 = local write "SetNr"(u8 0 ("SetNr")) -> ()
                n341 = call "PS35_PhaseInitTime.vi"("Axis number"=w381, "Control unit ID"=w379, "Value-In"=w380, "function"=TRUE ("WriteRead")) -> ()  [unwired: 4 in, 2 out]
              }
              frame 25 {
                n342 = local read "PhaseInitAmp"() -> (w385:i32)
                n343 = local read "AxisId"() -> (w386:i32)
                n344 = local read "Index"() -> (w384:i32)
                n345 = local write "SetNr"(u8 0 ("SetNr")) -> ()
                n346 = call "PS35_PhaseInitAmp.vi"("Axis number"=w386, "Control unit ID"=w384, "Value-In"=w385, "function"=TRUE ("WriteRead")) -> ()  [unwired: 4 in, 2 out]
              }
              frame 26 {
                n347 = local write "SetNr"(u8 0 ("SetNr")) -> ()
              }
              frame 27 {
                n348 = local read "MotorCommCounts"() -> (w391:i32)
                n349 = local read "AxisId"() -> (w392:i32)
                n350 = local read "Index"() -> (w390:i32)
                n351 = local write "SetNr"(u8 0 ("SetNr")) -> ()
                n352 = call "PS35_MotorCommCounts.vi"("Axis number"=w392, "Control unit ID"=w390, "Value-In"=w391, "function"=TRUE ("WriteRead")) -> ()  [unwired: 4 in, 2 out]
              }
              frame 28 {
                n353 = local read "AxisId"() -> (w397:i32)
                n354 = local read "EncLines"() -> (w396:i32)
                n355 = local read "Index"() -> (w395:i32)
                n356 = local write "SetNr"(u8 0 ("SetNr")) -> ()
                n357 = call "PS35_EncLines.vi"("Axis number"=w397, "Control unit ID"=w395, "Value-In"=w396, "function"=TRUE ("WriteRead")) -> ()  [unwired: 4 in, 2 out]
              }
            }
          }
        }
        n358 = case shown="True" w102 {
          frame False {
          }
          frame True {
            n359 = local write "SetNr"(u8 19 ("SetNr")) -> ()
          }
        }
        n360 = case shown="True" w89 {
          frame False {
          }
          frame True {
            n361 = local write "SetNr"(u8 23 ("SetNr")) -> ()
          }
        }
        n362 = case shown="True" w82 {
          frame False {
          }
          frame True {
            n363 = local write "SetNr"(u8 27 ("SetNr")) -> ()
          }
        }
        n364 = Not(x="End") -> (.not. x?=w161:bool)
      }
    }
  }
